vi "http 501 not implemented error.vi"(11 "application request in":T3) -> (3 "application request out":T1)   [LabVIEW 2016, in "Basic HTTPS server.lvclass"]
uses:
  Basic HTTPS server.lvclass
  http request.ctl
  http method.ctl
  HTTP headers/http header data.ctl
  http response.ctl
  HTTP headers/http headers.lvlib
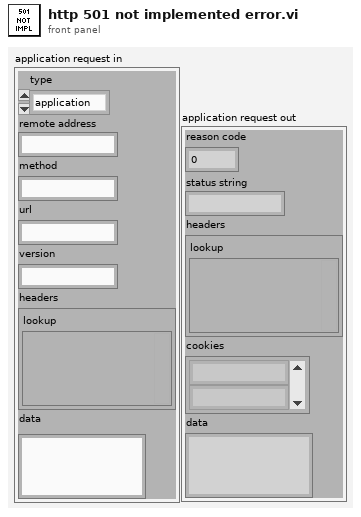
[diagram p1: front panel]
types:
  T1 = typedef "Basic HTTPS server.lvclass/http response.ctl" = cluster{"reason code":u16, "status string":string, "headers":T2, "cookies":string[], "data":string}
  T2 = typedef "http headers.lvlib/http header data.ctl" = cluster{"lookup":variant}
  T3 = typedef "Basic HTTPS server.lvclass/http request.ctl" = cluster{"type":T4, "remote address":string, "method":string, "url":string, "version":string, "headers":T2, "data":string}
  T4 = typedef "Basic HTTPS server.lvclass/http method.ctl" = enum16{"application", "error", "upgrade"}
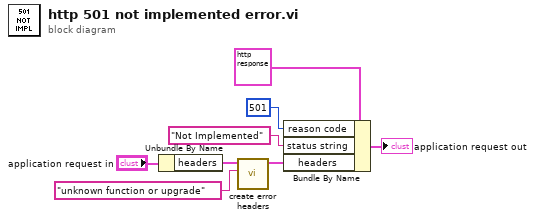
[diagram p0: block diagram]
diagram:
  n1 = Unbundle By Name("application request in") -> ("headers"=w1:T2)
  n2 = call "create error headers.vi"("custom error reason"="unknown function or upgrade", "headers in"=w1) -> ("headers out"=w3:T2)  [unwired: 9 in]
  n3 = Bundle By Name(cluster=T1 {"reason code"=0, "status string"="", "headers"={"lookup"=variant}, "cookies"=[], "data"=""} ("application request"), "reason code"=u16 501, "status string"="Not Implemented", "headers"=w3) -> (→"application request out":T1)
